vi "r3_placing_error.vi"() -> ()   [LabVIEW 2016]
uses:
  Classes/Controllers/Motion/Copy of Motion Folder/Motion.lvclass
  Classes/Controllers/Camera/Copy of Controller Folder/Controller.lvclass
panel:
  in  "Default sensor type B size":dbl[](array[numeric])=[22.0, 101.5, 78.448, -0.011805]
  in  "Default sensor type A size":dbl[](array[numeric])=[22.0, 129.5, 78.448, -0.011805]
  in  "Default HDI type A size":dbl[](array[numeric])=[24.3, 129.2, 78.448, -0.011805]
  in  "Default HDI type B size":dbl[](array[numeric])=[24.3, 101.2, 78.448, -0.011805]
  in  "Default sensor crossmark \nposition 2":dbl[](array[numeric])=[293.05283, 988.31451, 78.532999, -0.011805]
  in  "Default sensor crossmark \nposition 1":dbl[](array[numeric])=[293.10553, 1090.486, 78.527999, -0.011805]
  in  "Default HDI alignment \nmark position 2":dbl[](array[numeric])=[292.30667, 988.88691, 78.923999, -0.011805]
  in  "Default HDI alignment \nmark position":dbl[](array[numeric])=[292.37323, 1091.0515, 78.932996, -0.011805]
  out "Type B rotation error":dbl format="%#_8e"
  out "Type B Y error":dbl format="%#_8g"
  out "Type B X error":dbl format="%#_8g"
  out "Type A rotation error":dbl format="%#_8e"
  out "Type A Y error":dbl format="%#_8g"
  out "Type A X error":dbl format="%#_8g"
  out "HDI/sesnor array":bool[](array[boolean])
  out "type a/b array":bool[](array[boolean])
  in  "Type A/ Type B":bool
  in  "HDI / Sensor":bool
  out "the copy array":dbl[](array[numeric]) format="%#_8g"
  out "buttom right C":dbl[](array[numeric]) format="%#_8g"
  out "X position":dbl[](array[numeric]) format="%#_8g"
  out "Yposition":dbl[](array[numeric]) format="%#_8g"
  out "A C center point":dbl[](array[numeric]) format="%#_8g"
  out "loop counting":dbl
  out "rotation":dbl[](array[numeric]) format="%#_8g"
  in  "Stop":bool
  in  "DO measurement":bool=TRUE
  out "buttom left B":dbl[](array[numeric]) format="%#_8g"
  out "upper left A":dbl[](array[numeric]) format="%#_8g"
  out "r-phi":dbl[](array[numeric])
  out "A B center point":dbl[](array[numeric])
  # "HDI - Sensor = placing error"
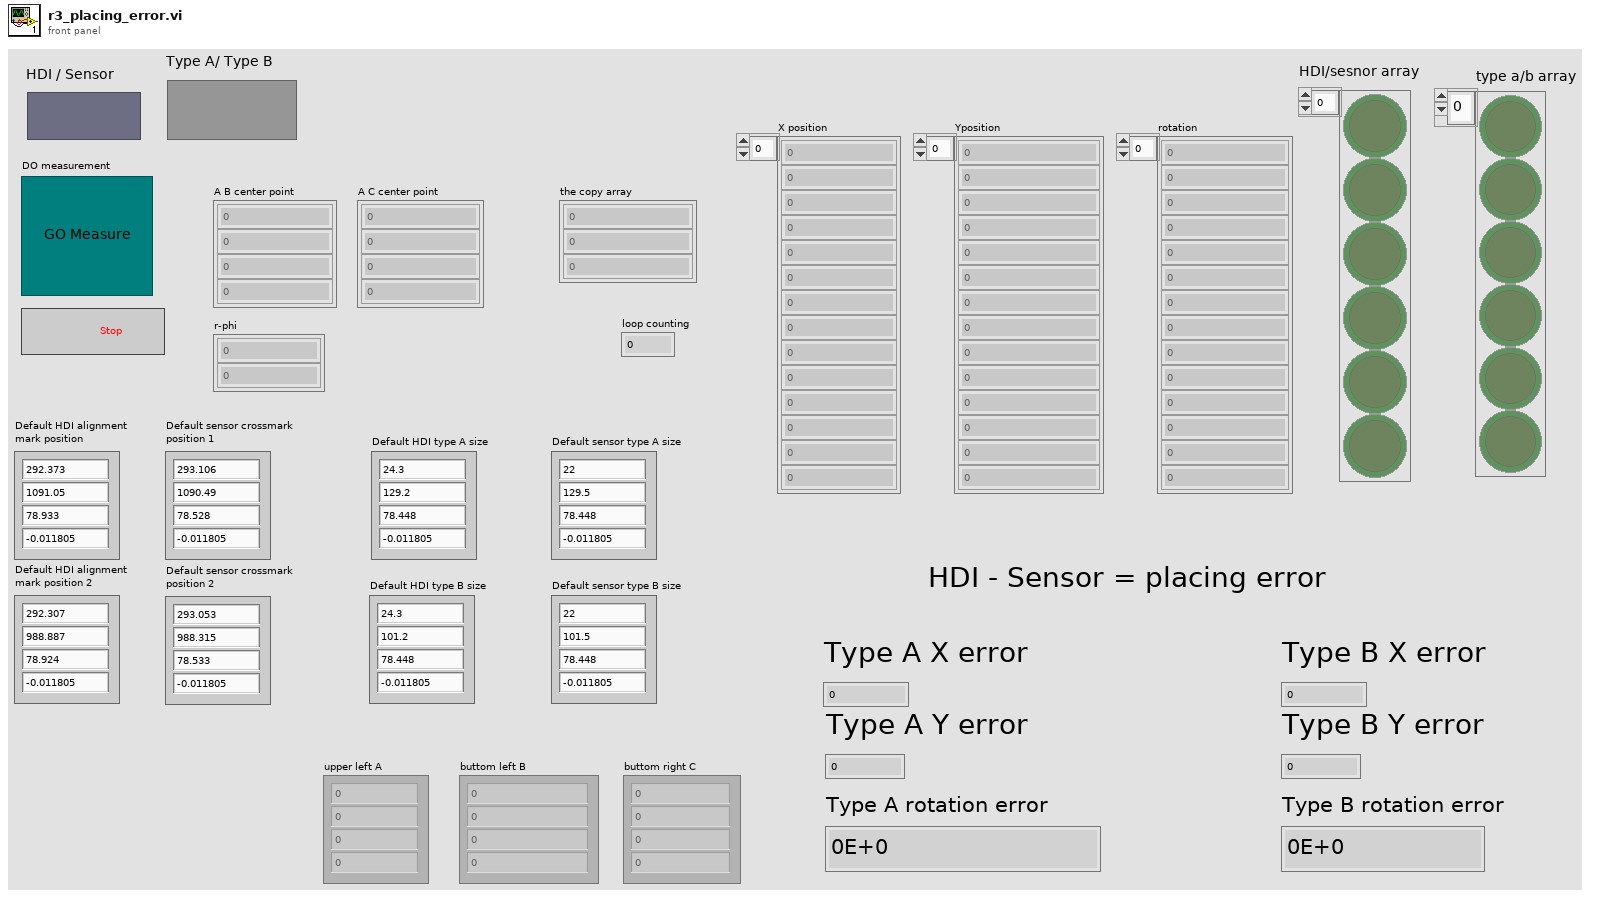
[diagram p1: front panel]
types:
  T1 = typedef "Controller.lvclass/Controllers.ctl" = cluster{"Copy of Motion.lvclass":refnum<class "Motion.lvclass">, "Copy of I-O.lvclass":refnum<class "I-O.lvclass">, "Copy of Dispenser.lvclass":refnum<class "Dispenser.lvclass">}
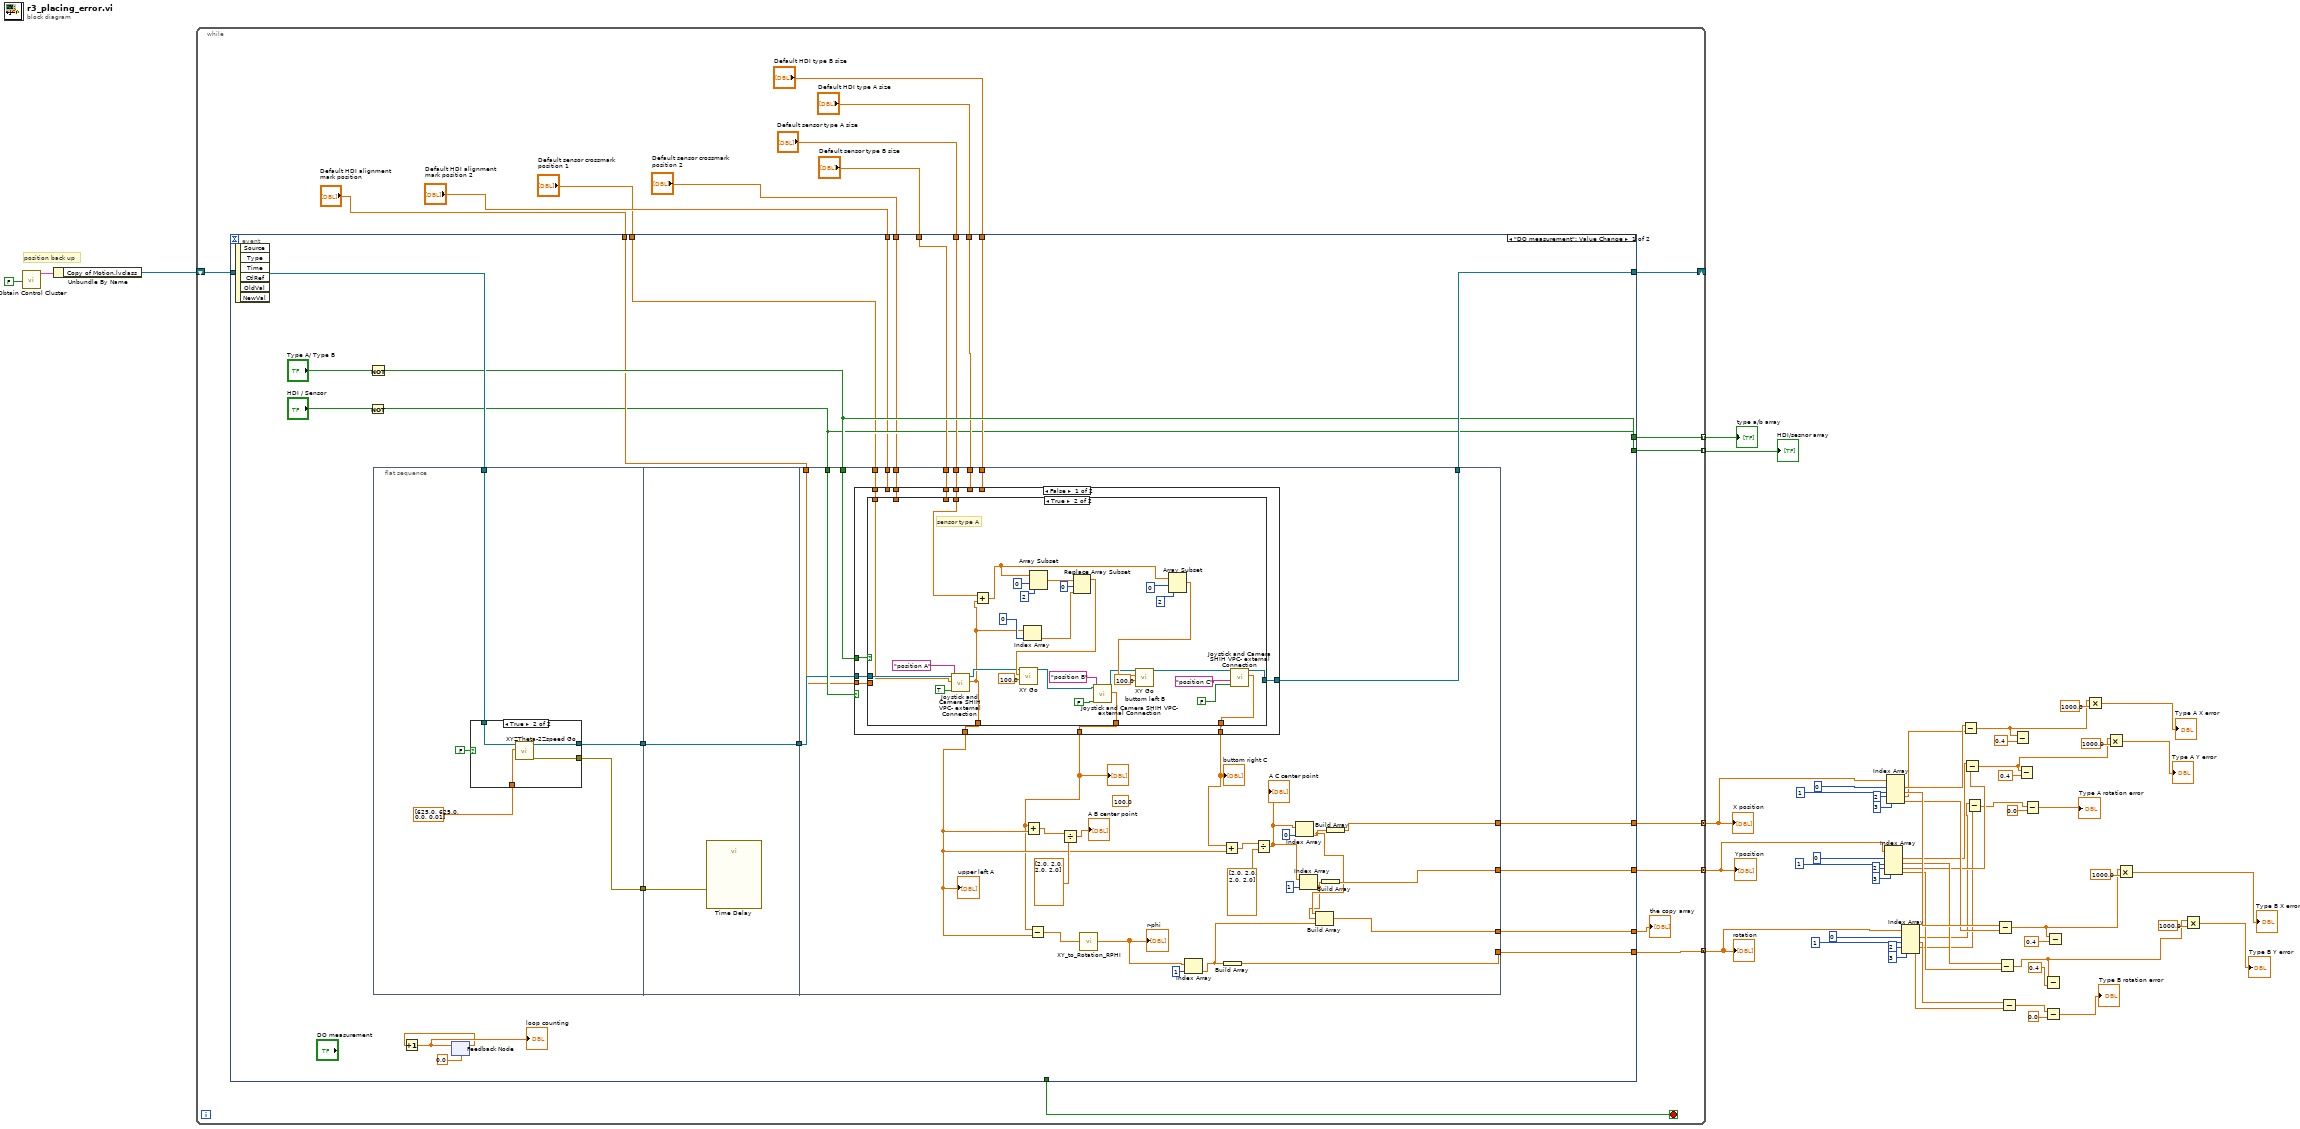
[diagram p0: block diagram]
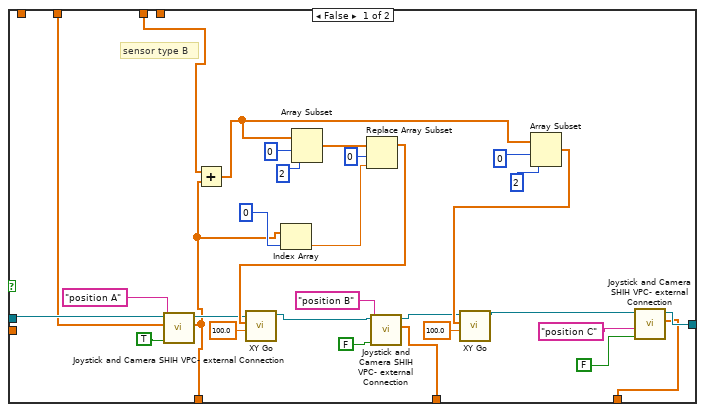
[diagram p3: hidden frame]
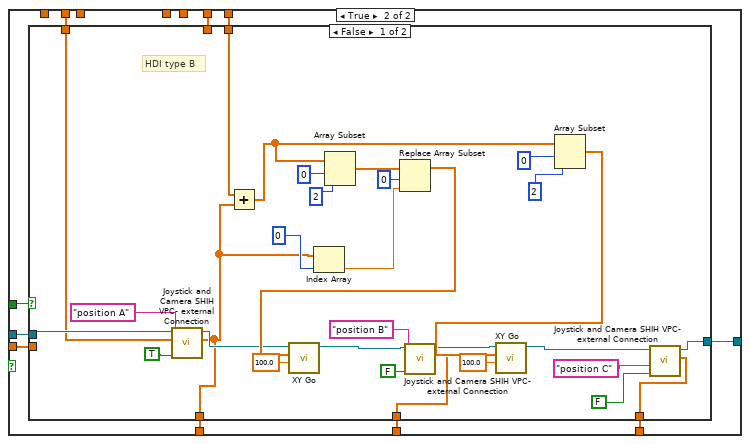
[diagram p4: hidden frame]
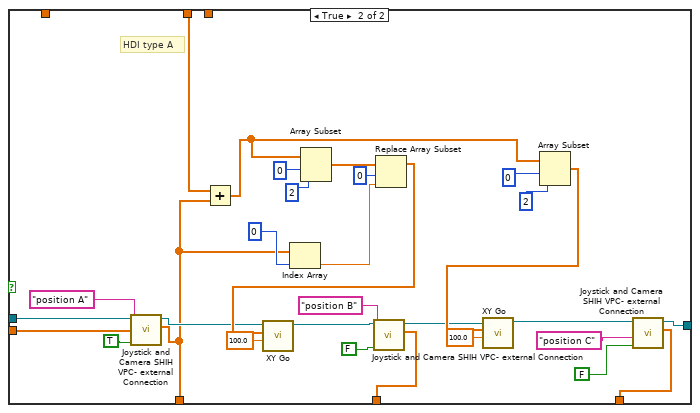
[diagram p5: hidden frame]
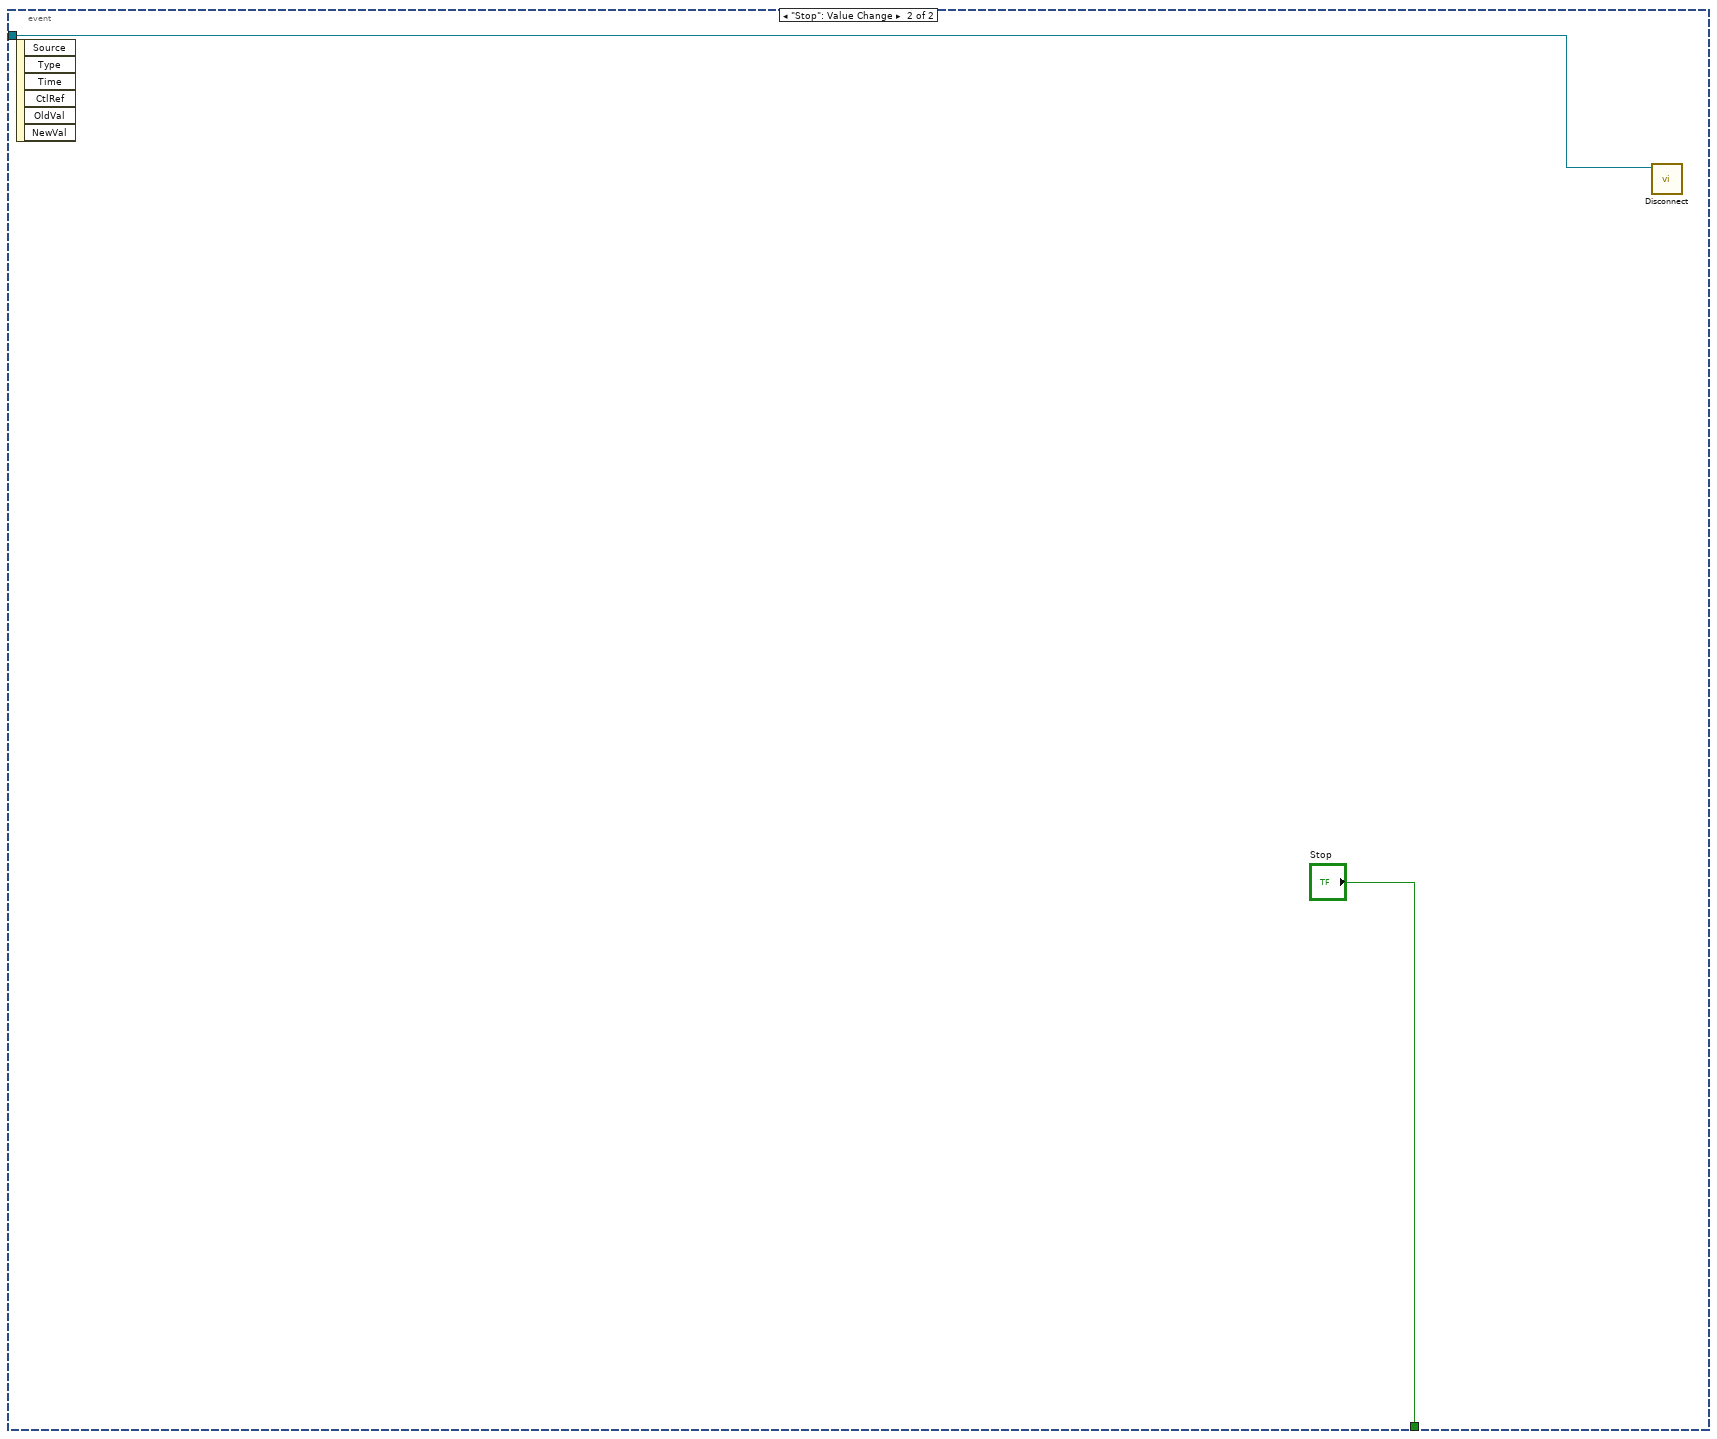
[diagram p6: hidden frame]
diagram:
  # "position back up"
  n1 = call "Obtain Control Cluster.vi"("I/O"=FALSE) -> ("Control Out"=w54:T1)  [unwired: 10 in]
  n2 = Unbundle By Name(w54) -> ("Copy of Motion.lvclass"=w52:refnum<class "Motion.lvclass">)
  n3 = while {
    shift-right: [w69] -> _
    shift-left: w52 -> [w71]
    tunnel: [w68] -> w35 mode=concatenating
    tunnel: [w67] -> w37 mode=concatenating
    tunnel: [w66] -> w36 mode=concatenating
    tunnel: [w64] -> w51 mode=indexing
    tunnel: [w63] -> w50 mode=indexing
    stop <- w70 stop-if-true
    n4 = event shown="[0] \"DO measurement\": Value Change" {
      selector: _ -> [_ _]
      dyn-events: _ -> [_ _]
      timeout: _ -> [_ _]
      tunnel: w71 -> [w95 w283]
      tunnel: [_ "Stop"] -> w70
      tunnel: [w93 _] -> w69
      tunnel: [w94 _] -> w68
      tunnel: [w89 _] -> w67
      tunnel: [w88 _] -> w66
      tunnel: [w87 _] -> w65
      tunnel: [w84 _] -> w64
      tunnel: [w78 _] -> w63
      tunnel: "Default HDI type A size" -> [w83 _]
      tunnel: "Default HDI type B size" -> [w82 _]
      tunnel: "Default sensor type A size" -> [w81 _]
      tunnel: "Default sensor type B size" -> [w80 _]
      tunnel: "Default HDI alignment \nmark position" -> [w79 _]
      tunnel: "Default HDI alignment \nmark position 2" -> [w74 _]
      tunnel: "Default sensor crossmark \nposition 1" -> [w73 _]
      tunnel: "Default sensor crossmark \nposition 2" -> [w72 _]
      event "DO measurement": Value Change {
        n5 = event-data() -> ()  [unwired: 1 in, 6 out]
        n6 = Not(x="HDI / Sensor") -> (.not. x?=w78:bool)
        n7 = Not(x="Type A/ Type B") -> (.not. x?=w84:bool)
        n8 = flat-sequence {
          tunnel: w95 -> [w99]
          tunnel: [w98] -> w77
          tunnel: [w97] -> w76
          tunnel: w77 -> [w107]
          tunnel: [w106] -> w75
          tunnel: w76 -> [w106]
          tunnel: w75 -> [w114]
          tunnel: [w134] -> w94
          tunnel: [w112] -> w93
          tunnel: [w128] -> w89
          tunnel: [w127] -> w88
          tunnel: [w123] -> w87
          tunnel: w78 -> [w122]
          tunnel: w84 -> [w121]
          tunnel: w83 -> [w120]
          tunnel: w82 -> [w119]
          tunnel: w81 -> [w117]
          tunnel: w80 -> [w116]
          tunnel: w79 -> [w113]
          tunnel: w74 -> [w110]
          tunnel: w73 -> [w109]
          tunnel: w72 -> [w108]
          frame #0 {
            n9 = case shown="True" FALSE {
              tunnel: dbl[] [625.0, 625.0, 0.0, 0.01] ("Parking position") -> [_ w105]
              tunnel: w99 -> [w101 w104]
              tunnel: [_ w103] -> w98
              tunnel: [w101 w102] -> w97
              frame False {
              }
              frame True {
                n10 = call "XYZTheta-2Zspeed Go.vi"("XYZTheta In"=w105, "Motion in"=w104) -> ("error out"=w103:errorcluster, "Motion out"=w102:refnum<class "Motion.lvclass">)  [unwired: 7 in, 1 out]
              }
            }
          }
          frame #1 {
            n11 = call "Time Delay"("error in (no error)"=w107) -> ()  [unwired: 10 in, 1 out]
          }
          frame #2 {
            (unwired) 100.0 ("Speed")
            n12 = case shown="False" w122 {
              tunnel: w121 -> [w151 w221]
              tunnel: w120 -> [_ w220]
              tunnel: w119 -> [_ w219]
              tunnel: [w146 w218] -> w118
              tunnel: w117 -> [w150 _]
              tunnel: w116 -> [w149 _]
              tunnel: [w145 w217] -> w115
              tunnel: w114 -> [w148 w216]
              tunnel: w113 -> [w147 w215]
              tunnel: [w143 w214] -> w112
              tunnel: [w144 w213] -> w111
              tunnel: w110 -> [_ w212]
              tunnel: w109 -> [w142 _]
              tunnel: w108 -> [w141 _]
              frame False {
                n13 = case shown="True" w151 {
                  tunnel: w150 -> [_ w203]
                  tunnel: w149 -> [w173 _]
                  tunnel: w148 -> [w166 w196]
                  tunnel: w147 -> [_ _]
                  tunnel: [w154 w184] -> w146
                  tunnel: [w161 w190] -> w145
                  tunnel: [w155 w186] -> w144
                  tunnel: [w156 w185] -> w143
                  tunnel: w142 -> [_ w182]
                  tunnel: w141 -> [w152 _]
                  frame False {
                    # "sensor type B"
                    n14 = call "Joystick and Camera SHIH VPC- external Connection.vi"("Motion in"=w166, "XYZTheta"=w152, "Measurement Point"="position A", "Inital GO"=TRUE) -> ("Motion out"=w165:refnum<class "Motion.lvclass">, "Sum"=w154:dbl[])  [unwired: 3 in, 2 out]
                    n15 = Add(x=w173, y=w154) -> (x+y=w178:dbl[])
                    n16 = Index Array(array=w154, index=0) -> (element=w153:dbl)
                    n17 = Array Subset(array=w178, index=0, length=2) -> (w179:dbl[])
                    n18 = Replace Array Subset(array=w179, new element=w153, index=0) -> (w172:dbl[])
                    n19 = call-dynamic "XY Go.vi"("Speed"=100.0, "XY"=w172, "Motion in"=w165) -> ("Motion out"=w162:refnum<class "Motion.lvclass">)  [unwired: 7 in, 1 out]
                    n20 = call "Joystick and Camera SHIH VPC- external Connection.vi"("Motion in"=w162, "Measurement Point"="position B", "Inital GO"=FALSE) -> ("Motion out"=w160:refnum<class "Motion.lvclass">, "Sum"=w161:dbl[])  [unwired: 4 in, 2 out]
                    n21 = Array Subset(array=w178, index=0, length=2) -> (w171:dbl[])
                    n22 = call-dynamic "XY Go.vi"("Speed"=100.0, "XY"=w171, "Motion in"=w160) -> ("Motion out"=w157:refnum<class "Motion.lvclass">)  [unwired: 7 in, 1 out]
                    n23 = call "Joystick and Camera SHIH VPC- external Connection.vi"("Motion in"=w157, "Measurement Point"="position C", "Inital GO"=FALSE) -> ("Motion out"=w156:refnum<class "Motion.lvclass">, "Sum"=w155:dbl[])  [unwired: 4 in, 2 out]
                  }
                  frame True {
                    # "sensor type A"
                    n24 = call "Joystick and Camera SHIH VPC- external Connection.vi"("Motion in"=w196, "XYZTheta"=w182, "Measurement Point"="position A", "Inital GO"=TRUE) -> ("Motion out"=w195:refnum<class "Motion.lvclass">, "Sum"=w184:dbl[])  [unwired: 3 in, 2 out]
                    n25 = Add(x=w203, y=w184) -> (x+y=w207:dbl[])
                    n26 = Index Array(array=w184, index=0) -> (element=w183:dbl)
                    n27 = Array Subset(array=w207, index=0, length=2) -> (w206:dbl[])
                    n28 = Replace Array Subset(array=w206, new element=w183, index=0) -> (w202:dbl[])
                    n29 = call-dynamic "XY Go.vi"("Speed"=100.0, "XY"=w202, "Motion in"=w195) -> ("Motion out"=w192:refnum<class "Motion.lvclass">)  [unwired: 7 in, 1 out]
                    n30 = call "Joystick and Camera SHIH VPC- external Connection.vi"("Motion in"=w192, "Measurement Point"="position B", "Inital GO"=FALSE) -> ("Motion out"=w191:refnum<class "Motion.lvclass">, "Sum"=w190:dbl[])  [unwired: 4 in, 2 out]
                    n31 = Array Subset(array=w207, index=0, length=2) -> (w201:dbl[])
                    n32 = call-dynamic "XY Go.vi"("Speed"=100.0, "XY"=w201, "Motion in"=w191) -> ("Motion out"=w187:refnum<class "Motion.lvclass">)  [unwired: 7 in, 1 out]
                    n33 = call "Joystick and Camera SHIH VPC- external Connection.vi"("Motion in"=w187, "Measurement Point"="position C", "Inital GO"=FALSE) -> ("Motion out"=w185:refnum<class "Motion.lvclass">, "Sum"=w186:dbl[])  [unwired: 4 in, 2 out]
                  }
                }
              }
              frame True {
                n34 = case shown="False" w221 {
                  tunnel: w220 -> [_ w273]
                  tunnel: w219 -> [w243 _]
                  tunnel: [w224 w258] -> w218
                  tunnel: [w231 w266] -> w217
                  tunnel: w216 -> [w235 w261]
                  tunnel: w215 -> [_ w260]
                  tunnel: [w226 w254] -> w214
                  tunnel: [w225 w252] -> w213
                  tunnel: w212 -> [w222 _]
                  frame False {
                    # "HDI type B"
                    n35 = call "Joystick and Camera SHIH VPC- external Connection.vi"("Motion in"=w235, "XYZTheta"=w222, "Measurement Point"="position A", "Inital GO"=TRUE) -> ("Motion out"=w236:refnum<class "Motion.lvclass">, "Sum"=w224:dbl[])  [unwired: 3 in, 2 out]
                    n36 = Add(x=w243, y=w224) -> (x+y=w247:dbl[])
                    n37 = Index Array(array=w224, index=0) -> (element=w223:dbl)
                    n38 = Array Subset(array=w247, index=0, length=2) -> (w246:dbl[])
                    n39 = Replace Array Subset(array=w246, new element=w223, index=0) -> (w242:dbl[])
                    n40 = call-dynamic "XY Go.vi"("Speed"=100.0, "XY"=w242, "Motion in"=w236) -> ("Motion out"=w233:refnum<class "Motion.lvclass">)  [unwired: 7 in, 1 out]
                    n41 = call "Joystick and Camera SHIH VPC- external Connection.vi"("Motion in"=w233, "Measurement Point"="position B", "Inital GO"=FALSE) -> ("Motion out"=w232:refnum<class "Motion.lvclass">, "Sum"=w231:dbl[])  [unwired: 4 in, 2 out]
                    n42 = Array Subset(array=w247, index=0, length=2) -> (w241:dbl[])
                    n43 = call-dynamic "XY Go.vi"("Speed"=100.0, "XY"=w241, "Motion in"=w232) -> ("Motion out"=w227:refnum<class "Motion.lvclass">)  [unwired: 7 in, 1 out]
                    n44 = call "Joystick and Camera SHIH VPC- external Connection.vi"("Motion in"=w227, "Measurement Point"="position C", "Inital GO"=FALSE) -> ("Motion out"=w226:refnum<class "Motion.lvclass">, "Sum"=w225:dbl[])  [unwired: 4 in, 2 out]
                  }
                  frame True {
                    # "HDI type A"
                    n45 = call "Joystick and Camera SHIH VPC- external Connection.vi"("Motion in"=w261, "XYZTheta"=w260, "Measurement Point"="position A", "Inital GO"=TRUE) -> ("Motion out"=w259:refnum<class "Motion.lvclass">, "Sum"=w258:dbl[])  [unwired: 3 in, 2 out]
                    n46 = Add(x=w273, y=w258) -> (x+y=w277:dbl[])
                    n47 = Index Array(array=w258, index=0) -> (element=w272:dbl)
                    n48 = Array Subset(array=w277, index=0, length=2) -> (w276:dbl[])
                    n49 = Replace Array Subset(array=w276, new element=w272, index=0) -> (w271:dbl[])
                    n50 = call-dynamic "XY Go.vi"("Speed"=100.0, "XY"=w271, "Motion in"=w259) -> ("Motion out"=w265:refnum<class "Motion.lvclass">)  [unwired: 7 in, 1 out]
                    n51 = call "Joystick and Camera SHIH VPC- external Connection.vi"("Motion in"=w265, "Measurement Point"="position B", "Inital GO"=FALSE) -> ("Motion out"=w264:refnum<class "Motion.lvclass">, "Sum"=w266:dbl[])  [unwired: 4 in, 2 out]
                    n52 = Array Subset(array=w277, index=0, length=2) -> (w270:dbl[])
                    n53 = call-dynamic "XY Go.vi"("Speed"=100.0, "XY"=w270, "Motion in"=w264) -> ("Motion out"=w255:refnum<class "Motion.lvclass">)  [unwired: 7 in, 1 out]
                    n54 = call "Joystick and Camera SHIH VPC- external Connection.vi"("Motion in"=w255, "Measurement Point"="position C", "Inital GO"=FALSE) -> ("Motion out"=w254:refnum<class "Motion.lvclass">, "Sum"=w252:dbl[])  [unwired: 4 in, 2 out]
                  }
                }
              }
            }
            "upper left A" <- w118
            "buttom left B" <- w115
            "buttom right C" <- w111
            n55 = Add(x=w115, y=w118) -> (x+y=w137:dbl[])
            n56 = Subtract(x=w115, y=w118) -> (x-y=w140:dbl[])
            n57 = Divide(x=w137, y=dbl[] [2.0, 2.0, 2.0, 2.0]) -> (x/y=→"A B center point":dbl[])
            n58 = call "XY_to_Rotation_RPHI.vi"("X-Y"=w140) -> ("r-phi"=w135:dbl[])
            "r-phi" <- w135
            n59 = Index Array(array=w135, index=1) -> (element=w124:dbl)
            n60 = Add(x=w111, y=w118) -> (x+y=w132:dbl[])
            n61 = Build Array(w124) -> (w134:dbl[])
            n62 = Divide(x=w132, y=dbl[] [2.0, 2.0, 2.0, 2.0]) -> (x/y=w129:dbl[])
            "A C center point" <- w129
            n63 = Index Array(array=w129, index=0) -> (element=w126:dbl)
            n64 = Index Array(array=w129, index=1) -> (element=w125:dbl)
            n65 = Build Array(w126, w125, w124) -> (w123:dbl[])
            n66 = Build Array(w125) -> (w127:dbl[])
            n67 = Build Array(w126) -> (w128:dbl[])
          }
        }
        n68 = feedback #1(0.0) -> (w90:dbl)
        n69 = Increment(x=w90) -> (x+1=w92:dbl)
        "loop counting" <- w92
        n70 = feedback-in #1(w92) -> ()
      }
      event "Stop": Value Change {
        n71 = event-data() -> ()  [unwired: 1 in, 6 out]
        n72 = call-dynamic "Disconnect.vi"("Controller in"=w283) -> ()  [unwired: 9 in, 1 out]
      }
    }
    "the copy array" <- w65
  }
  "rotation" <- w35
  "X position" <- w37
  "Yposition" <- w36
  "type a/b array" <- w51
  "HDI/sesnor array" <- w50
  n73 = Index Array(array=w36, index #1=0 ("index"), index #2=1 ("index"), index #3=2 ("index"), index #4=3 ("index")) -> (element #1=w30:dbl, element #2=w29:dbl, element #3=w28:dbl, element #4=w27:dbl)
  n74 = Index Array(array=w37, index #1=0 ("index"), index #2=1 ("index"), index #3=2 ("index"), index #4=3 ("index")) -> (element #1=w34:dbl, element #2=w33:dbl, element #3=w32:dbl, element #4=w31:dbl)
  n75 = Index Array(array=w35, index #1=0 ("index"), index #2=1 ("index"), index #3=2 ("index"), index #4=3 ("index")) -> (element #1=w26:dbl, element #2=w25:dbl, element #3=w24:dbl, element #4=w23:dbl)
  n76 = Subtract(x=w34, y=w32) -> (x-y=w2:dbl)
  n77 = Subtract(x=w30, y=w28) -> (x-y=w1:dbl)
  n78 = Subtract(x=w26, y=w24) -> (x-y=w16:dbl)
  n79 = Subtract(x=w33, y=w31) -> (x-y=w4:dbl)
  n80 = Subtract(x=w29, y=w27) -> (x-y=w3:dbl)
  n81 = Subtract(x=w25, y=w23) -> (x-y=w15:dbl)
  n82 = Subtract(x=w2, y=0.4) -> ()  [unwired: 1 out]
  n83 = Subtract(x=w1, y=0.4) -> ()  [unwired: 1 out]
  n84 = Subtract(x=w16, y=0.0) -> (x-y=→"Type A rotation error":dbl)
  n85 = Subtract(x=w3, y=0.4) -> ()  [unwired: 1 out]
  n86 = Subtract(x=w15, y=0.0) -> (x-y=→"Type B rotation error":dbl)
  n87 = Subtract(x=w4, y=0.4) -> ()  [unwired: 1 out]
  n88 = Multiply(x=w2, y=1000.0) -> (x*y=→"Type A X error":dbl)
  n89 = Multiply(x=w1, y=1000.0) -> (x*y=→"Type A Y error":dbl)
  n90 = Multiply(x=w4, y=1000.0) -> (x*y=→"Type B X error":dbl)
  n91 = Multiply(x=w3, y=1000.0) -> (x*y=→"Type B Y error":dbl)
